vi "AMC Multiple Targets Example 2 (RT).vi"() -> ()   [LabVIEW 2017]
panel:
  in  "Exit":bool
  out "Process":bool
  out "Status":string
  in  "State Variables":cluster{"CurrentFile":path}
  # "Target2"
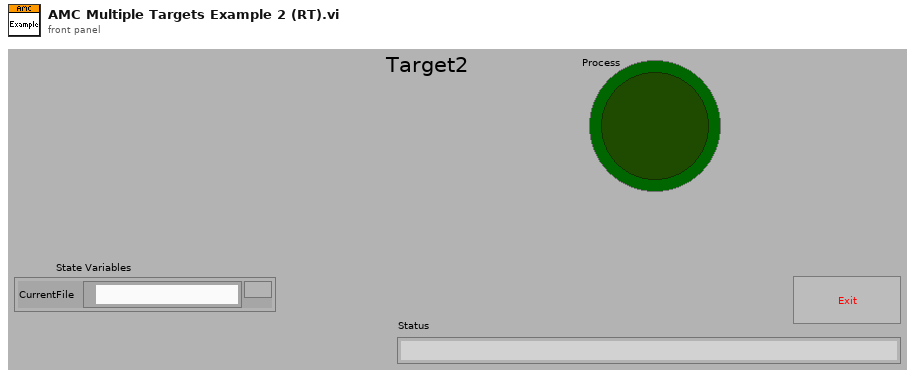
[diagram p1: front panel]
types:
  T1 = typedef "amc_Message Queue.ctl" = refnum<queue>
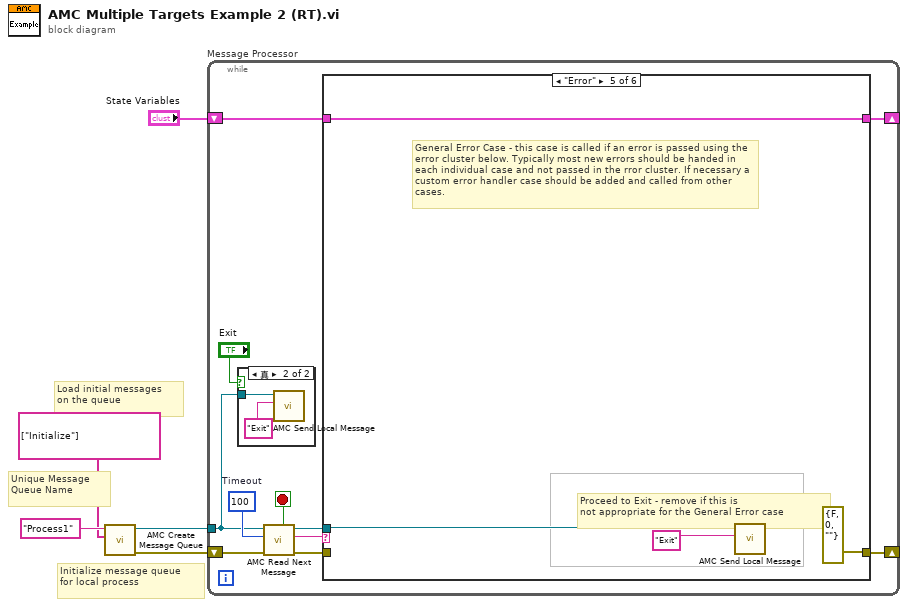
[diagram p0: block diagram]
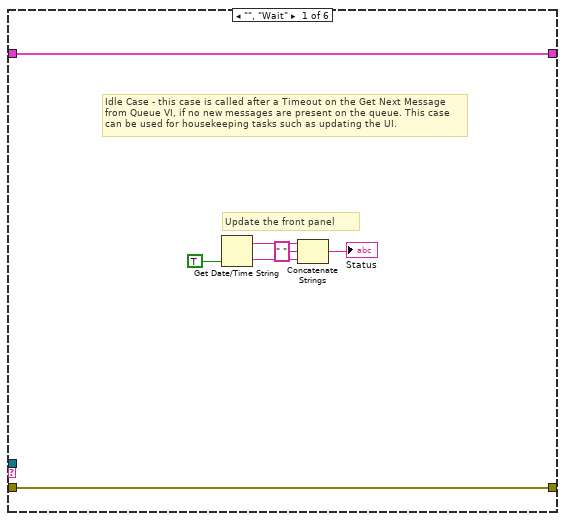
[diagram p3: hidden frame]
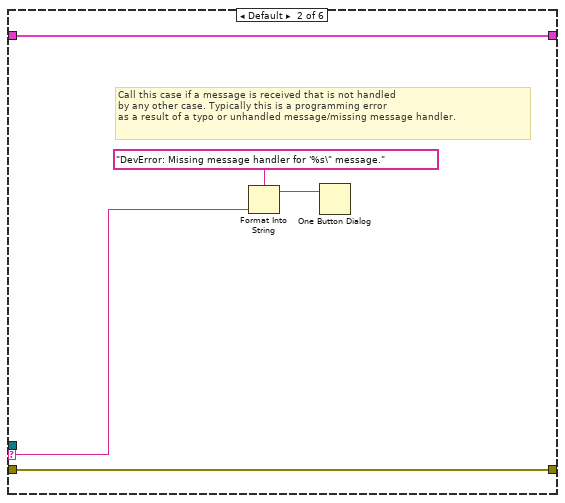
[diagram p4: hidden frame]
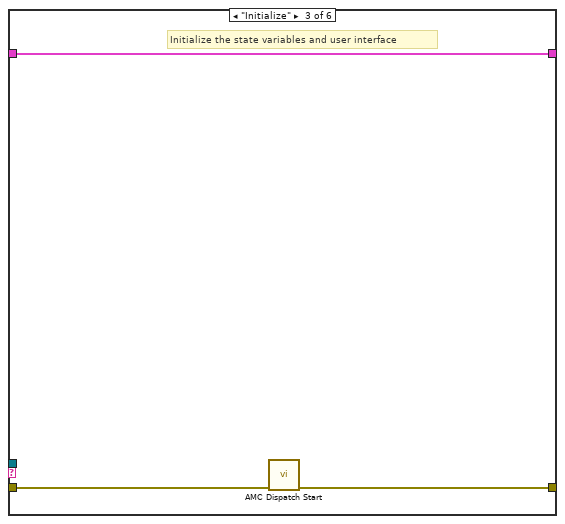
[diagram p5: hidden frame]
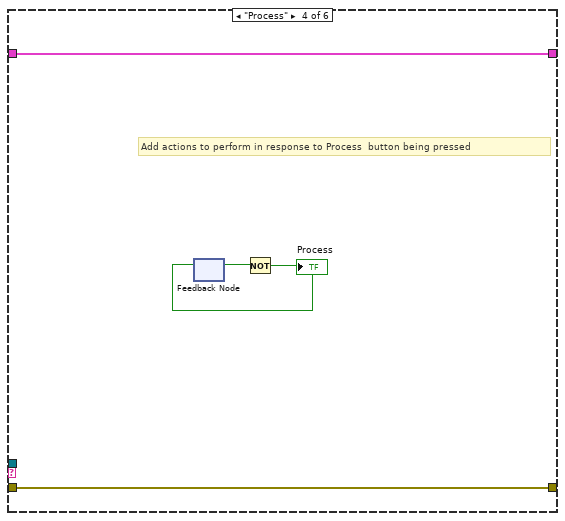
[diagram p6: hidden frame]
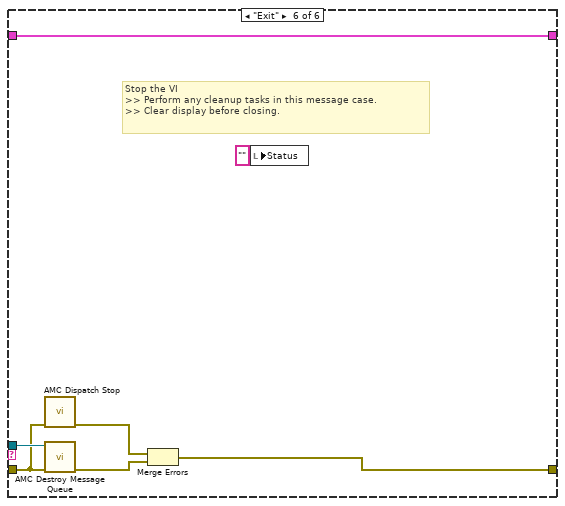
[diagram p7: hidden frame]
diagram:
  # "Initialize message queue\nfor local process"
  # "Unique Message\nQueue Name"
  # "Load initial messages\non the queue"
  n1 = call "AMC Create Message Queue.vi"("Initial Message Names"=string[] ["Initialize"], "Message Queue Name"="Process1" ("Message queue name (unnamed)")) -> ("error out"=w2:errorcluster, "Message Queue out"=w4:T1)  [unwired: 3 in, 5 out]
  n2 = while "Message Processor" {
    shift-left: w2 -> [w11]
    shift-right: [w12] -> _
    tunnel: w4 -> [w6]
    shift-left: "State Variables" -> [w16]
    shift-right: [w15] -> _
    stop <- w8 stop-if-true
    w10 = 100  # Timeout
    n3 = case shown="真" "Exit" {
      tunnel: w6 -> [_ w17]
      frame False {
      }
      frame True {
        n4 = call "AMC Send Local Message.vi"("Message Name"="Exit", "Message Queue in"=w17) -> ()  [unwired: 4 in, 6 out]
      }
    }
    n5 = call "AMC Read Next Message.vi"("error in (no error)"=w11, "timeout (1ms)"=w10, "Message Queue in"=w6) -> ("error out"=w13:errorcluster, "Message Name"=w9:string, "Message Queue out"=w14:T1, "Exit Process"=w8:bool)  [unwired: 1 in, 4 out]
    n6 = case shown="\"Error\"" w9 {
      selector: w9 -> [_ w28 _ _ _ _]
      tunnel: [w25 w30 w33 w36 w41 w48] -> w15
      tunnel: w16 -> [w25 w30 w33 w36 w41 w48]
      tunnel: w14 -> [_ _ _ _ w39 w46]
      tunnel: w13 -> [w24 w29 w32 w37 _ w42]
      tunnel: [w24 w29 w31 w37 errorcluster {"status"=FALSE, "code"=0, "source"=""} ("error out") w43] -> w12
      frame "", "Wait" {
        # "Update the front panel"
        # "Idle Case - this case is called after a Timeout on the Get Next Message from Queue VI, if no new messages are present on the queue. This case can be used for housekeeping tasks such as updating the UI."
        n7 = Get Date/Time String(want seconds? (F)=TRUE) -> (date string=w23:string, time string=w22:string)  [unwired: 2 out]
        n8 = Concatenate Strings(w23, " " ("string"), w22) -> (→"Status":string)
      }
      frame Default {
        # "Call this case if a message is received that is not handled \nby any other case. Typically this is a programming error\nas a result of a typo or unhandled message/missing message handler."
        n9 = Format Into String(format string="DevError: Missing message handler for '%s\" message." ("message"), w28) -> (resulting string=w26:string)  [unwired: 2 in, 1 out]
        n10 = One Button Dialog(message=w26) -> ()  [unwired: 2 out]
      }
      frame "Initialize" {
        # "Initialize the state variables and user interface"
        n11 = call "AMC Dispatch Start.vi"("error in (no error)"=w32) -> ("error out"=w31:errorcluster)  [unwired: 1 in, 9 out]
      }
      frame "Process" {
        # "Add actions to perform in response to Process  button being pressed"
        n12 = feedback #1() -> (w35:bool)  [unwired: 1 out]
        n13 = Not(x=w35) -> (.not. x?=w34:bool)
        "Process" <- w34
        n14 = feedback-in #1(w34) -> ()
      }
      frame "Error" {
        # "Proceed to Exit - remove if this is\nnot appropriate for the General Error case"
        # "General Error Case - this case is called if an error is passed using the error cluster below. Typically most new errors should be handed in each individual case and not passed in the rror cluster. If necessary a custom error handler case should be added and called from other cases."
        n15 = call "AMC Send Local Message.vi"("Message Name"="Exit", "Message Queue in"=w39) -> ()  [unwired: 4 in, 6 out]
      }
      frame "Exit" {
        # "Stop the VI\n>> Perform any cleanup tasks in this message case.\n>> Clear display before closing."
        n16 = call "AMC Dispatch Stop.vi"("error in (no error)"=w42) -> ("error out"=w44:errorcluster)  [unwired: 10 out]
        n17 = call "AMC Destroy Message Queue.vi"("error in (no error)"=w42, "Message Queue in"=w46) -> ("error out"=w45:errorcluster)  [unwired: 9 out]
        n18 = Merge Errors(w44, w45) -> (w43:errorcluster)
        n19 = local write "Status"("" ("Status")) -> ()
      }
    }
  }
